vi "SetBiasAH2700.vi"(8 "error in (no error)":errorcluster, 9 "Bias (Off)":i32(ring) items=["Disabled", "100 megohm", "1 megohm"], 10 "V/A ?":enum16{"DC V"}(ring), 11 "On/Off":bool) -> (0 "error out":errorcluster)   [LabVIEW 2018]
uses:
  Instance           1 15Saved   SetBias .vi
  Instance           2 15Saved   SetBias .vi
  Equipment/Capacity_Bridge_AH2700A/Andeen-Hagerling 2700/Andeen-Hagerling 2700.lvlib
panel:
  # "On: Bias einschalten\nOff: Bias ausschalten"
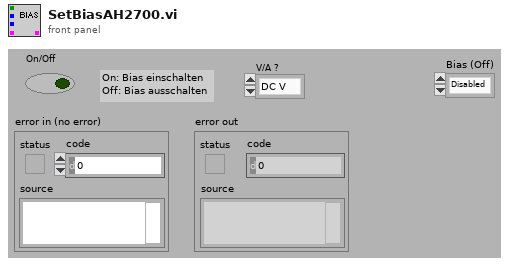
[diagram p1: front panel]
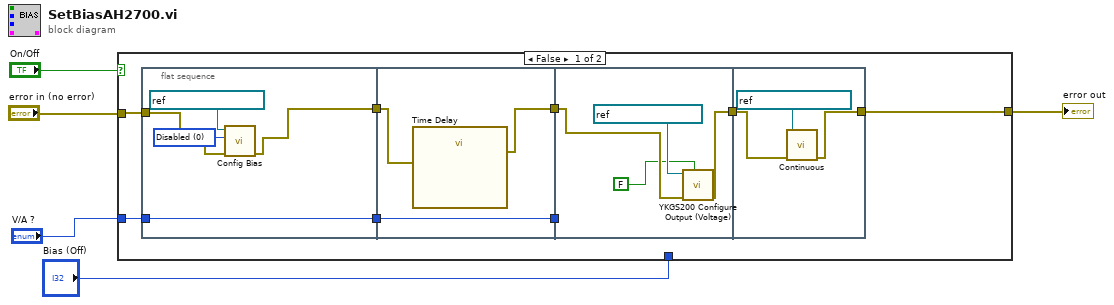
[diagram p0: block diagram]
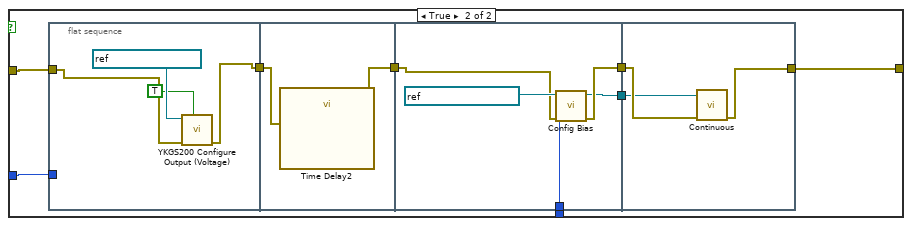
[diagram p2: hidden frame]
diagram:
  n1 = case shown="False" "On/Off" {
    tunnel: "error in (no error)" -> [w12 w36]
    tunnel: "V/A ?" -> [w13 w35]
    tunnel: [w9 w30] -> w2
    tunnel: "Bias (Off)" -> [_ w29]
    frame False {
      n2 = flat-sequence {
        tunnel: w13 -> [w18]
        tunnel: w12 -> [w17]
        tunnel: [w16] -> w11
        tunnel: [w18] -> w7
        tunnel: w11 -> [w21]
        tunnel: [w20] -> w10
        tunnel: [w19] -> w8
        tunnel: w7 -> [w19]
        tunnel: w10 -> [w24]
        tunnel: w8 -> [_]
        tunnel: [w23] -> w6
        tunnel: [w27] -> w9
        tunnel: w6 -> [w28]
        frame #0 {
          w14 = 0 items=["Disabled", "100 megohm", "1 megohm"] ("Bias (Off)")
          n3 = call "Config Bias.vi"("error in"=w17, "Bias (Off)"=w14, "VISA resource name"=refnum<visa-resource-name> "GPIB0::28::INSTR") -> ("error out"=w16:errorcluster)  [unwired: 7 in, 1 out]
        }
        frame #1 {
          n4 = call "Time Delay"("error in (no error)"=w21) -> ("error out"=w20:errorcluster)  [unwired: 10 in]
        }
        frame #2 {
          n5 = call "YKGS200 Configure Output (Voltage).vi"("Enable Output (T: Enable)"=FALSE, "error in (no error)"=w24, "VISA resource name"=refnum<visa-resource-name> "GPIB0::6::INSTR") -> ("error out"=w23:errorcluster)  [unwired: 7 in, 1 out]
        }
        frame #3 {
          n6 = call "Continuous.vi"("error in"=w28, "VISA resource name"=refnum<visa-resource-name> "GPIB0::28::INSTR") -> ("error out"=w27:errorcluster)  [unwired: 8 in, 1 out]
        }
      }
    }
    frame True {
      n7 = flat-sequence {
        tunnel: w36 -> [w40]
        tunnel: w35 -> [_]
        tunnel: [w39] -> w34
        tunnel: w34 -> [w42]
        tunnel: [w41] -> w33
        tunnel: w33 -> [w46]
        tunnel: [w45] -> w32
        tunnel: [w44] -> w31
        tunnel: w29 -> [w43]
        tunnel: w32 -> [w50]
        tunnel: w31 -> [w49]
        tunnel: [w48] -> w30
        frame #0 {
          n8 = call "YKGS200 Configure Output (Voltage).vi"("Enable Output (T: Enable)"=TRUE, "error in (no error)"=w40, "VISA resource name"=refnum<visa-resource-name> "GPIB0::6::INSTR") -> ("error out"=w39:errorcluster)  [unwired: 7 in, 1 out]
        }
        frame #1 {
          n9 = call "Time Delay2"("error in (no error)"=w42) -> ("error out"=w41:errorcluster)  [unwired: 10 in]
        }
        frame #2 {
          n10 = call "Config Bias.vi"("error in"=w46, "Bias (Off)"=w43, "VISA resource name"=refnum<visa-resource-name> "GPIB0::28::INSTR") -> ("error out"=w45:errorcluster, "VISA resource name out"=w44:refnum<visa-resource-name>)  [unwired: 7 in]
        }
        frame #3 {
          n11 = call "Continuous.vi"("error in"=w50, "VISA resource name"=w49) -> ("error out"=w48:errorcluster)  [unwired: 8 in, 1 out]
        }
      }
    }
  }
  "error out" <- w2
